vi "Validate CLI Arguments.vi"(8 "error in":errorcluster, 10 "CLI Arguments Setting":T1, 11 "Command":string) -> (0 "error out":errorcluster)   [LabVIEW 2025]
doc: "This VI validates that every CLI command receives the necessary arguments."
uses:
  Type Definitions/CLI Argument Setting--cluster.ctl
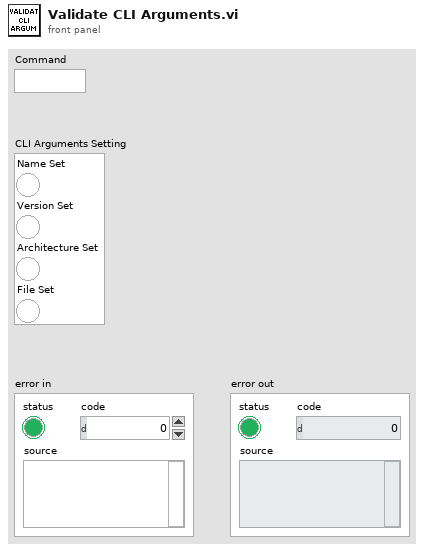
[diagram p1: front panel]
types:
  T1 = typedef "CLI Argument Setting--cluster.ctl" = cluster{"Name Set":bool, "Version Set":bool, "Architecture Set":bool, "File Set":bool}
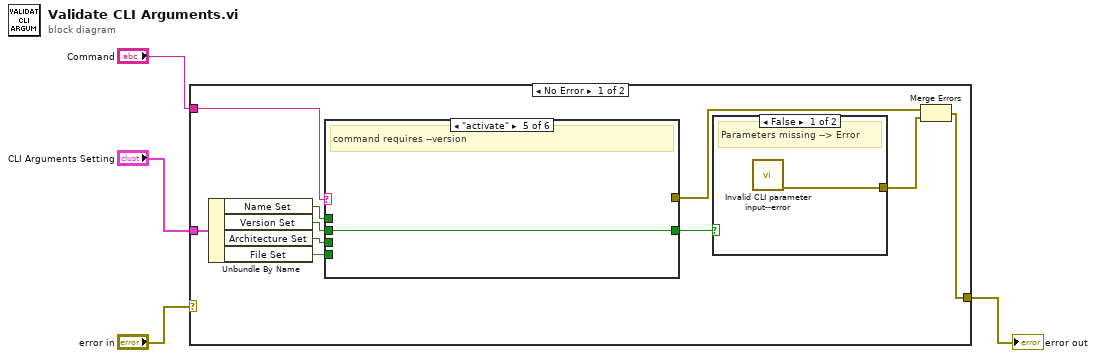
[diagram p0: block diagram]
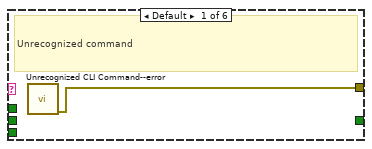
[diagram p3: hidden frame]
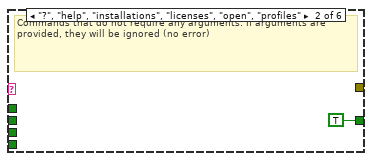
[diagram p4: hidden frame]
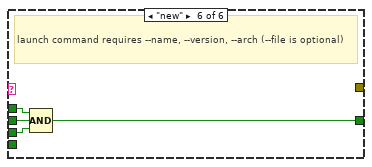
[diagram p7: hidden frame]
diagram:
  n1 = case shown="No Error" "error in" {
    selector: "error in" -> [_ w25]
    tunnel: [w12 w25] -> w4
    tunnel: "Command" -> [w10 _]
    tunnel: "CLI Arguments Setting" -> [w9 _]
    frame No Error {
      n2 = Unbundle By Name(w9) -> ("Name Set"=w7:bool, "Version Set"=w6:bool, "Architecture Set"=w5:bool, "File Set"=w8:bool)
      n3 = case shown="\"activate\"" w10 {
        tunnel: [_ TRUE w18 w19 w20 w21] -> w11
        tunnel: [w16 _ _ _ _ _] -> w13
        tunnel: w7 -> [_ _ w18 _ _ w24]
        tunnel: w6 -> [_ _ _ _ w20 w22]
        tunnel: w5 -> [_ _ _ _ _ w23]
        tunnel: w8 -> [_ _ _ w19 _ _]
        frame Default {
          # "Unrecognized command"
          n4 = call "Unrecognized CLI Command--error.vi"() -> ("error out"=w16:errorcluster)  [unwired: 11 in]
        }
        frame "?", "help", "installations", "licenses", "open", "profiles" {
          # "Commands that do not require any arguments. If arguments are provided, they will be ignored (no error)"
        }
        frame "delete", "launch" {
          # "launch/delete command requires --name"
        }
        frame "set-file" {
          # "command requires --file"
        }
        frame "activate" {
          # "command requires --version"
        }
        frame "new" {
          # "launch command requires --name, --version, --arch (--file is optional)"
          n5 = Compound Arithmetic op=AND(w24, w22, w23) -> (w21:bool)
        }
      }
      n6 = case shown="False" w11 {
        tunnel: [w15 _] -> w14
        frame False {
          # "Parameters missing --> Error"
          n7 = call "Invalid CLI parameter input--error.vi"() -> ("error out"=w15:errorcluster)  [unwired: 11 in]
        }
        frame True {
          # "all parameters were provided"
        }
      }
      n8 = Merge Errors(w13, w14) -> (w12:errorcluster)
    }
    frame Error {
      # "Pass error without further action."
    }
  }
  "error out" <- w4
